vi "Initialize.vi"() -> (0 "SmartScope out":refnum<k24>)   [LabVIEW 2013]
uses:
  C:/Program Files (x86)/LabNation/SmartScope/DeviceInterface.dll
  Program Files (x86)/LabNation/SmartScope/DeviceInterface.dll
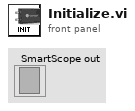
[diagram p1: front panel]
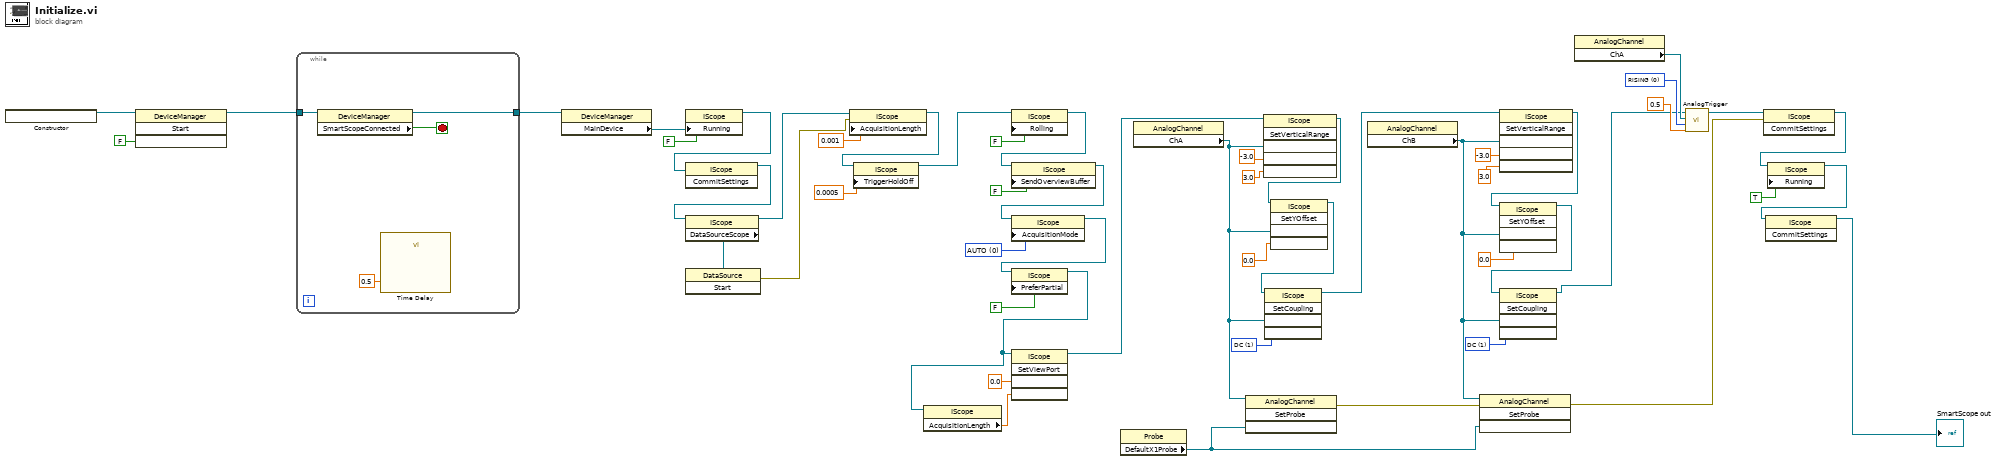
[diagram p0: block diagram]
diagram:
  w45 = 0 items=["RISING", "FALLING", "ANY"] ("edge")
  w43 = 1 items=["AC", "DC"] ("coupling")
  w37 = 1 items=["AC", "DC"] ("coupling")
  w32 = 0 items=["AUTO", "NORMAL", "SINGLE"] ("AcquisitionMode")
  n1 = constructor class="DeviceManager"() -> (reference out=w14:refnum<k24>)  [unwired: 3 in, 2 out]
  n2 = invoke class="DeviceManager" method="Start"(reference=w14, FALSE ("async")) -> (reference out=w15:refnum<k24>)  [unwired: 2 in, 3 out]
  n3 = while {
    tunnel: w15 -> [w56]
    tunnel: [w55] -> w17
    stop <- w54 stop-if-true
    n4 = property class="DeviceManager"(reference=w56) -> (reference out=w55:refnum<k24>, "SmartScopeConnected"=w54:bool)  [unwired: 1 in, 1 out]
    n5 = call "Time Delay"(10:0.5 ("Delay Time (s)")) -> ()  [unwired: 10 in, 1 out]
  }
  n6 = property class="DeviceManager"(reference=w17) -> ("MainDevice"=w18:refnum<k24>)  [unwired: 1 in, 2 out]
  n7 = property class="IScope"(reference=w18, "Running"=FALSE) -> (reference out=w20:refnum<k24>)  [unwired: 1 in, 1 out]
  n8 = invoke class="IScope" method="CommitSettings"(reference=w20) -> (reference out=w28:refnum<k24>)  [unwired: 2 in, 2 out]
  n9 = property class="IScope"(reference=w28) -> (reference out=w53:refnum<k24>, "DataSourceScope"=w29:refnum<k24>)  [unwired: 1 in, 1 out]
  n10 = invoke class="DataSource" method="Start"(reference=w29) -> (error out=w50:errorcluster)  [unwired: 2 in, 2 out]
  n11 = property class="IScope"(reference=w53, error in=w50, "AcquisitionLength"=0.001) -> (reference out=w23:refnum<k24>)  [unwired: 1 out]
  n12 = property class="IScope"(reference=w23, "TriggerHoldOff"=0.0005 ("AcquisitionLength")) -> (reference out=w24:refnum<k24>)  [unwired: 1 in, 1 out]
  n13 = property class="IScope"(reference=w24, "Rolling"=FALSE ("LogicAnalyserEnabled")) -> (reference out=w25:refnum<k24>)  [unwired: 1 in, 1 out]
  n14 = property class="IScope"(reference=w25, "SendOverviewBuffer"=FALSE) -> (reference out=w26:refnum<k24>)  [unwired: 1 in, 1 out]
  n15 = property class="IScope"(reference=w26, "AcquisitionMode"=w32) -> (reference out=w27:refnum<k24>)  [unwired: 1 in, 1 out]
  n16 = property class="IScope"(reference=w27, "PreferPartial"=FALSE) -> (reference out=w35:refnum<k24>)  [unwired: 1 in, 1 out]
  n17 = property class="IScope"(reference=w35) -> ("AcquisitionLength"=w36:dbl)  [unwired: 1 in, 2 out]
  n18 = invoke class="IScope" method="SetViewPort"(reference=w35, 0.0 ("offset"), w36) -> (reference out=w13:refnum<k24>)  [unwired: 2 in, 4 out]
  n19 = property class="Probe"() -> ("DefaultX1Probe"=w4:refnum<k24>)  [unwired: 2 in, 2 out]
  n20 = property class="AnalogChannel"() -> ("ChA"=w6:refnum<k24>)  [unwired: 2 in, 2 out]
  n21 = invoke class="AnalogChannel" method="SetProbe"(reference=w6, w4) -> (error out=w2:errorcluster)  [unwired: 2 in, 3 out]
  n22 = invoke class="IScope" method="SetVerticalRange"(reference=w13, w6, sgl -3.0 ("minimum"), sgl 3.0 ("maximum")) -> (reference out=w10:refnum<k24>)  [unwired: 2 in, 5 out]
  n23 = invoke class="IScope" method="SetYOffset"(reference=w10, w6, sgl 0.0 ("offset")) -> (reference out=w8:refnum<k24>)  [unwired: 2 in, 4 out]
  n24 = invoke class="IScope" method="SetCoupling"(reference=w8, w6, w37) -> (reference out=w7:refnum<k24>)  [unwired: 2 in, 4 out]
  n25 = property class="AnalogChannel"() -> ("ChB"=w3:refnum<k24>)  [unwired: 2 in, 2 out]
  n26 = invoke class="AnalogChannel" method="SetProbe"(reference=w3, error in=w2, w4) -> (error out=w1:errorcluster)  [unwired: 1 in, 3 out]
  n27 = invoke class="IScope" method="SetVerticalRange"(reference=w7, w3, sgl -3.0 ("minimum"), sgl 3.0 ("maximum")) -> (reference out=w40:refnum<k24>)  [unwired: 2 in, 5 out]
  n28 = invoke class="IScope" method="SetYOffset"(reference=w40, w3, sgl 0.0 ("offset")) -> (reference out=w42:refnum<k24>)  [unwired: 2 in, 4 out]
  n29 = invoke class="IScope" method="SetCoupling"(reference=w42, w3, w43) -> (reference out=w5:refnum<k24>)  [unwired: 2 in, 4 out]
  n30 = property class="AnalogChannel"() -> ("ChA"=w44:refnum<k24>)  [unwired: 2 in, 2 out]
  n31 = call "AnalogTrigger.vi"(1:sgl 0.5 ("level"), 2:w45, 3:w44, 4:w5) -> (0:w52:refnum<k24>)
  n32 = invoke class="IScope" method="CommitSettings"(reference=w52, error in=w1) -> (reference out=w49:refnum<k24>)  [unwired: 1 in, 2 out]
  n33 = property class="IScope"(reference=w49, "Running"=TRUE) -> (reference out=w48:refnum<k24>)  [unwired: 1 in, 1 out]
  n34 = invoke class="IScope" method="CommitSettings"(reference=w48) -> (reference out=→"SmartScope out":refnum<k24>)  [unwired: 2 in, 2 out]
